vi "Gear_Rail.vi"(0 "MotorControlDevRef":T4={"DeviceStatus"={"status"=FALSE, "code"=0, "source"=""}, "Type"=enum."PWM", "PWM"={"PWM Channel"=enum."Invalid", "DeadBand"={"Name"="", "maxPositivePwm"=0, "minPositivePwm"=0, "centerPwm"=0, "maxNegativePwm"=0, "minNegativePwm"=0, "angularRange"=0}}, "CAN"={"Device Number"=0, "SetOutput VI Ref"=variant(refnum<vi> refnum), "GetOutput VI Ref"=variant(refnum<vi> refnum), "Enable VI Ref"=variant(refnum<vi> refnum), "Disable VI Ref"=variant(refnum<vi> refnum), "Data"=variant}, "Invert"=FALSE}, 1 "dt_In_PID":dbl=-1.0 format="%.3f", 2 "Potentiometer_Input":dbl, 3 "Potentiometer_WantedPos":dbl(slide) scale=0.0..30.0, 4 "Motor_Input":dbl, 5 "Rail Parameters":T1={"Scale Positions"={"Forward_StartScale"=0.0, "Reverse_StartScale"=0.0, "Forward_Limit"=0.0, "Reverse_Limit"=0.0}, "Motor_Limit"=0.6, "Invert?"=FALSE, "PID gains"={"proportional gain (Kc)"=1.0, "integral time (Ti, min)"=0.01, "derivative time (Td, min)"=0.0}, "Timeout (ms)"=2000} {"PID gains"."derivative time (Td, min)" format="%.3f"; "PID gains"."integral time (Ti, min)" format="%.3f"; "PID gains"."proportional gain (Kc)" format="%.3f"}) -> (20 "dt_Out_PID":dbl format="%.3f")   [LabVIEW 2016]
uses:
  <vilib>/Rock Robotics/WPI/MotorControl/WPI_MotorControlDeviceRef.ctl
  <vilib>/Rock Robotics/WPI/MotorControl/WPI_MotorControlType.ctl
  <vilib>/Rock Robotics/SystemInterfaces/DIO/FPGA_DIOPWMChannel.ctl
  <vilib>/Rock Robotics/WPI/PWM/WPI_PWMDeadband.ctl
  TypeDefs/RailParameters_Type.ctl
  TypeDefs/MotorLimitPositions_Type.ctl
  Global_Var-RefNum/Global_Var_Other.vi
  <vilib>/addons/control/pid/pid.llb/PID (DBL).vi
  <vilib>/addons/control/pid/NI_PID_pid.lvlib
panel:
  out "Waveform Chart":T3(graph)
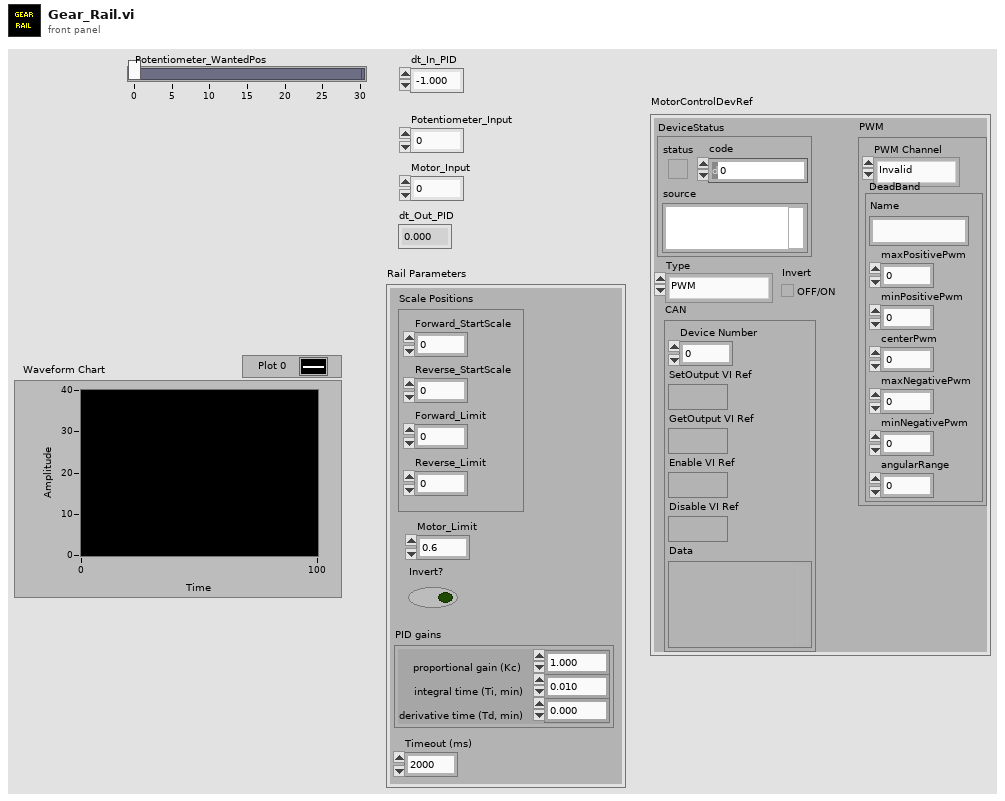
[diagram p1: front panel]
types:
  T1 = typedef "RailParameters_Type.ctl" = cluster{"Scale Positions":T2, "Motor_Limit":dbl, "Invert?":bool, "PID gains":cluster{"proportional gain (Kc)":dbl, "integral time (Ti, min)":dbl, "derivative time (Td, min)":dbl}, "Timeout (ms)":u32}
  T2 = typedef "MotorLimitPositions_Type.ctl" = cluster{"Forward_StartScale":dbl, "Reverse_StartScale":dbl, "Forward_Limit":dbl, "Reverse_Limit":dbl}
  T3 = cluster{"Potentiometer_Input":dbl, "Potentiometer_WantedPos":dbl}
  T4 = typedef "WPI_MotorControlDeviceRef.ctl" = cluster{"DeviceStatus":errorcluster, "Type":T5, "PWM":cluster{"PWM Channel":T6, "DeadBand":T7}, "CAN":cluster{"Device Number":u8, "SetOutput VI Ref":variant, "GetOutput VI Ref":variant, "Enable VI Ref":variant, "Disable VI Ref":variant, "Data":variant}, "Invert":bool}
  T5 = typedef "WPI_MotorControlType.ctl" = enum16{"PWM", "CAN"}
  T6 = typedef "FPGA_DIOPWMChannel.ctl" = enum8{"PWM 0", "PWM 1", "PWM 2", "PWM 3", "PWM 4", "PWM 5", "PWM 6", "PWM 7", "PWM 8", "PWM 9", "PWM MXP 0", "PWM MXP 1", "PWM MXP 2", "PWM MXP 3", "PWM MXP 4", "PWM MXP 5", "PWM MXP 6", "PWM MXP 7", "PWM MXP 8", "PWM MXP 9", "Invalid"}
  T7 = typedef "WPI_PWMDeadband.ctl" = cluster{"Name":string, "maxPositivePwm":i32, "minPositivePwm":i32, "centerPwm":i32, "maxNegativePwm":i32, "minNegativePwm":i32, "angularRange":u16}
  T8 = cluster{"proportional gain (Kc)":dbl, "integral time (Ti, min)":dbl, "derivative time (Td, min)":dbl}
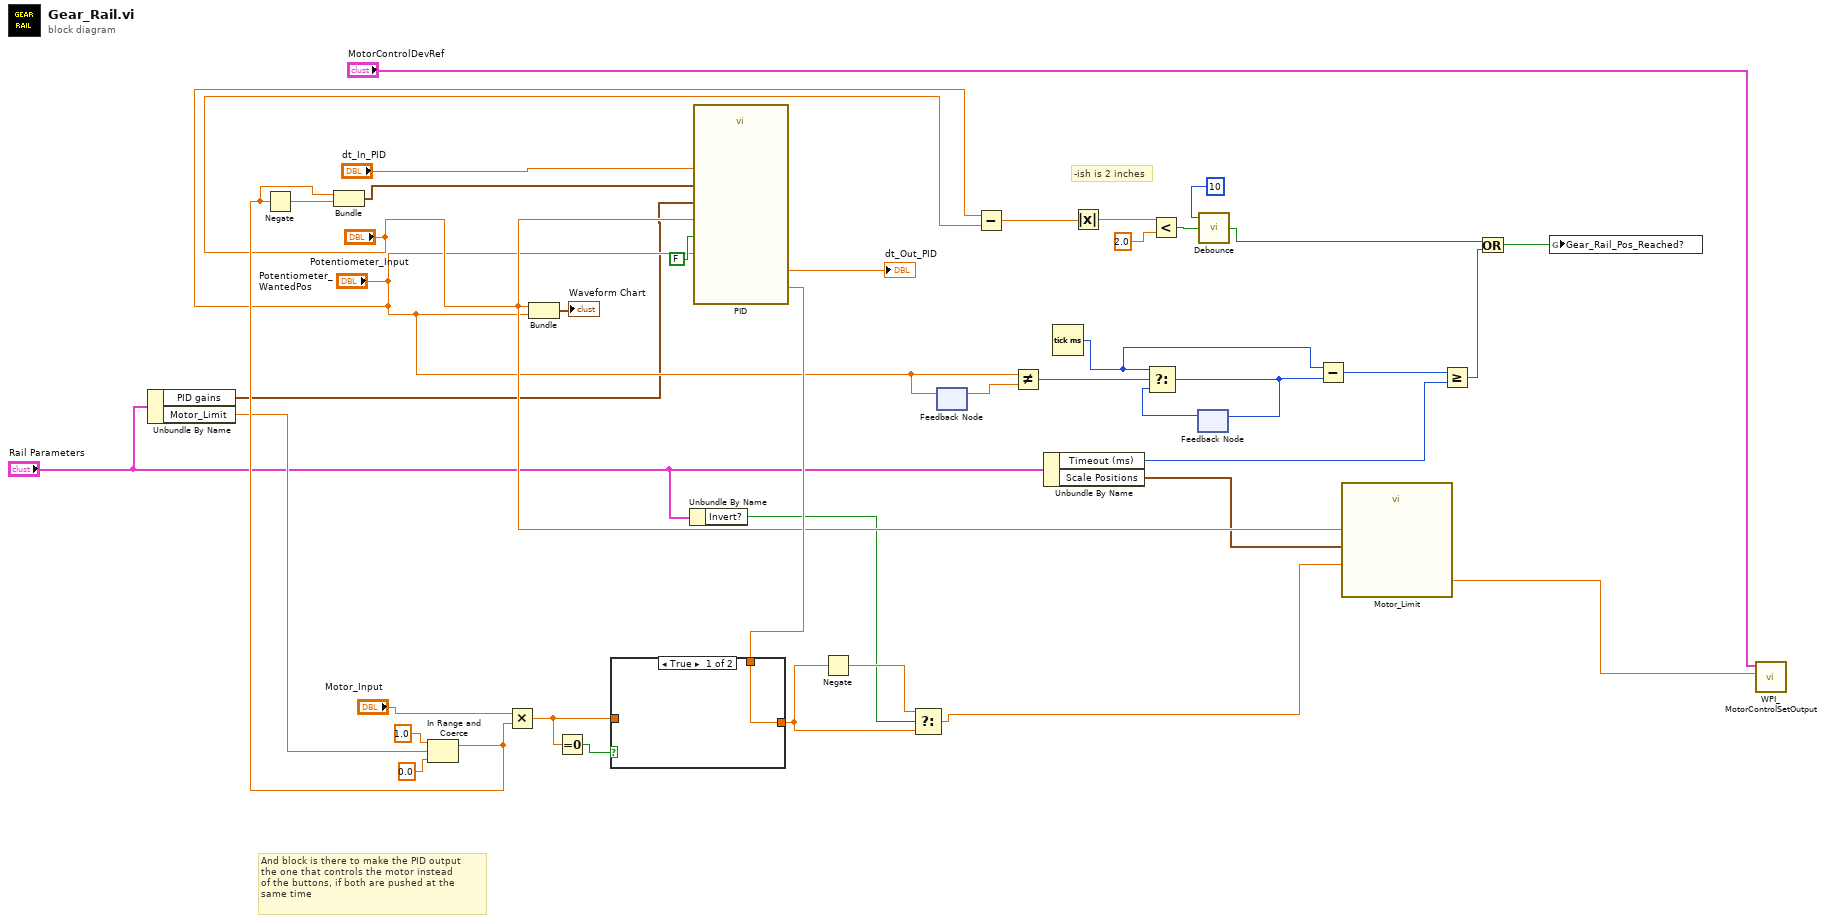
[diagram p0: block diagram]
diagram:
  # "-ish is 2 inches"
  # "And block is there to make the PID output \nthe one that controls the motor instead\nof the buttons, if both are pushed at the \nsame time"
  n1 = Unbundle By Name("Rail Parameters") -> ("PID gains"=w6:T8, "Motor_Limit"=w5:dbl)
  n2 = In Range and Coerce(upper limit=1.0, x=w5, lower limit=0.0) -> (coerced(x)=w19:dbl)  [unwired: 1 out]
  n3 = Negate(x=w19) -> (-x=w23:dbl)
  n4 = Bundle("upper limit"=w19, w23) -> (w22:cluster{"upper limit":dbl, dbl})  [unwired: 1 in]
  n5 = Multiply(x="Motor_Input", y=w19) -> (x*y=w25:dbl)
  n6 = Bundle("Potentiometer_Input"="Potentiometer_Input", "Potentiometer_WantedPos"="Potentiometer_WantedPos") -> (→"Waveform Chart":T3)  [unwired: 1 in]
  n7 = Equal To 0?(x=w25) -> (x = 0?=w24:bool)
  n8 = Unbundle By Name("Rail Parameters") -> ("Invert?"=w4:bool)
  n9 = call-poly <vilib>:"PID.vi"("reinitialize? (F)"=FALSE, "output range"=w22, "dt (s)"="dt_In_PID", "PID gains"=w6, "process variable"="Potentiometer_Input", "setpoint"="Potentiometer_WantedPos") -> ("dt out (s)"=→"dt_Out_PID":dbl, "output"=w31:dbl)  [unwired: 4 in]
  n10 = case shown="True" w24 {
    tunnel: [w41 w42] -> w38
    tunnel: w31 -> [w41 _]
    tunnel: w25 -> [_ w42]
    frame True {
    }
    frame False {
    }
  }
  n11 = Negate(x=w38) -> (-x=w40:dbl)
  n12 = Select(t=w40, s=w4, f=w38) -> (s? t:f=w27:dbl)
  n13 = feedback-in #1("Potentiometer_WantedPos") -> ()
  n14 = feedback #1() -> (w16:dbl)  [unwired: 1 in]
  n15 = Subtract(x="Potentiometer_WantedPos", y="Potentiometer_Input") -> (x-y=w32:dbl)
  n16 = Not Equal?(x="Potentiometer_WantedPos", y=w16) -> (x != y?=w14:bool)
  n17 = Unbundle By Name("Rail Parameters") -> ("Timeout (ms)"=w2:u32, "Scale Positions"=w1:T2)
  n18 = Tick Count (ms)() -> (millisecond timer value=w11:u32)
  n19 = Absolute Value(x=w32) -> (abs(x)=w33:dbl)
  n20 = Less?(x=w33, y=2.0) -> (x < y?=w30:bool)
  n21 = feedback #2() -> (w13:u32)  [unwired: 1 in]
  n22 = Select(t=w11, s=w14, f=w13) -> (s? t:f=w12:u32)
  n23 = feedback-in #2(w12) -> ()
  n24 = call "Debounce.vi"("Input"=w30, "Num samples"=10) -> ("Output"=w7:bool)  [unwired: 1 in]
  n25 = Subtract(x=w11, y=w12) -> (x-y=w10:u32)
  n26 = call "Motor_Limit.vi"("Current_Pos"="Potentiometer_Input", "Motor_Speed"=w27, "Scale Positions"=w1) -> ("New_Motor_Speed"=w28:dbl)  [unwired: 16 in]
  n27 = Greater Or Equal?(x=w10, y=w2) -> (x >= y?=w8:bool)
  n28 = Or(x=w7, y=w8) -> (x .or. y?=w9:bool)
  n29 = global write "Global_Var_Other.vi" "Gear_Rail_Pos_Reached?"(w9) -> ()
  n30 = call <vilib>:"WPI_MotorControlSetOutput.vi"("Output"=w28, "MotorControlDevRef"="MotorControlDevRef") -> ()  [unwired: 7 in, 3 out]
